vi "test_read-nmea-data2.vi"() -> ()   [LabVIEW 2019] (continued)
32,154,14,19,51,157,,6*69\n\t\n15:14:47.48\tF9P\t$GPGSV,3,3,09,25,12,306,,6*5B\n\t\n15:14:47.50\tF9P\t$GLGSV,2,1,08,69,10,031,33,70,70,037,27,71,54,207,28,72,05,210,,1*75\n\t\n15:14:47.52\tF9P\t$GLGSV,2,2,08,77,01,324,,84,19,123,21,85,69,072,36,86,38,331,,1*75\n\t\n15:14:47.54\tF9P\t$GLGSV,2,1,08,69,10,031,20,70,70,037,,71,54,207,24,72,05,210,,3*7C\n\t\n15:14:47.56\tF9P\t$GLGSV,2,2,08,77,01,324,,84,19,123,27,85,69,072,25,86,38,331,,3*73\n\t\n15:14:47.58\tF9P\t$GAGSV,2,1,08,02,08,296,09,04,67,115,26,09,33,193,34,11,72,001,24,7*75\n\t\n15:14:47.60\tF9P\t$GAGSV,2,2,08,12,39,103,28,19,25,045,35,25,08,248,21,36,27,309,18,7*73\n\t\n15:14:47.62\tF9P\t$GAGSV,2,1,08,02,08,296,,04,67,115,24,09,33,193,,11,72,001,,2*7A\n\t\n15:14:47.64\tF9P\t$GAGSV,2,2,08,12,39,103,,19,25,045,,25,08,248,,36,27,309,,2*70\n\t\n15:14:47.66\tF9P\t$GBGSV,2,1,06,07,,,24,11,48,133,32,14,87,101,26,28,,,26,1*7E\n\t\n15:14:47.68\tF9P\t$GBGSV,2,2,06,33,62,220,30,34,,,40,1*44\n\t\n15:14:47.70\tF9P\t$GBGSV,1,1,03,11,48,133,25,14,87,101,,33,62,220,,3*43\n\t\n15:14:47.72\tF9P\t$GNGLL,3723.60420,N,12656.96638,E,061449.00,A,A*78\n\t\n15:14:47.74\tF9P\t\t\n15:14:47.76\tF9P\t\t\n15:14:47.78\tF9P\t\t\n15:14:47.80\tF9P\t\t\n15:14:47.82\tF9P\t\t\n15:14:47.84\tF9P\t\t\n15:14:47.86\tF9P\t\t\n15:14:47.88\tF9P\t\t\n15:14:47.90\tF9P\t\t\n15:14:47.92\tF9P\t\t\n15:14:47.94\tF9P\t\t\n15:14:47.96\tF9P\t\t\n15:14:47.98\tF9P\t\t\n15:14:48.00\tF9P\t\t\n15:14:48.02\tF9P\t\t\n15:14:48.04\tF9P\t\t\n15:14:48.06\tF9P\t\t\n15:14:48.08\tF9P\t\t\n15:14:48.10\tF9P\t\t\n15:14:48.12\tF9P\t\t\n15:14:48.14\tF9P\t\t\n15:14:48.16\tF9P\t\t\n15:14:48.18\tF9P\t\t\n15:14:48.20\tF9P\t\t\n15:14:48.22\tF9P\t\t\n15:14:48.24\tF9P\t$GNRMC,061450.00,A,3723.60390,N,12656.96564,E,2.579,234.40,250720,,,A,V*01\n\t\n15:14:48.26\tF9P\t$GNVTG,234.40,T,,M,2.579,N,4.776,K,A*29\n\t\n15:14:48.28\tF9P\t$GNGGA,061450.00,3723.60390,N,12656.96564,E,1,12,0.64,46.4,M,18.5,M,,*78\n\t\n15:14:48.30\tF9P\t$GNGSA,A,3,12,06,19,05,17,09,04,02,,,,,1.14,0.64,0.95,1*0A\n\t\n15:14:48.32\tF9P\t$GNGSA,A,3,85,70,71,84,,,,,,,,,1.14,0.64,0.95,2*08\n\t\n15:14:48.34\tF9P\t$GNGSA,A,3,36,19,11,04,09,12,,,,,,,1.14,0.64,0.95,3*0A\n\t\n15:14:48.36\tF9P\t$GNGSA,A,3,14,11,33,,,,,,,,,,1.14,0.64,0.95,4*0B\n\t\n15:14:48.38\tF9P\t$GPGSV,3,1,09,02,56,320,22,04,17,043,37,05,38,248,32,06,64,051,35,1*69\n\t\n15:14:48.40\tF9P\t$GPGSV,3,2,09,09,44,073,41,12,23,276,25,17,32,154,28,19,51,157,32,1*61\n\t\n15:14:48.42\tF9P\t$GPGSV,3,3,09,25,12,306,15,1*58\n\t\n15:14:48.44\tF9P\t$GPGSV,3,1,09,02,56,320,,04,17,043,23,05,38,248,17,06,64,051,27,6*6F\n\t\n15:14:48.46\tF9P\t$GPGSV,3,2,09,09,44,073,27,12,23,276,16,17,32,154,14,19,51,157,,6*68\n\t\n15:14:48.48\tF9P\t$GPGSV,3,3,09,25,12,306,,6*5B\n\t\n15:14:48.50\tF9P\t$GLGSV,2,1,08,69,10,031,28,70,70,037,27,71,54,207,32,72,05,210,,1*74\n\t\n15:14:48.52\tF9P\t$GLGSV,2,2,08,77,01,324,,84,19,123,21,85,69,072,35,86,38,331,,1*76\n\t\n15:14:48.54\tF9P\t$GLGSV,2,1,08,69,10,031,20,70,70,037,,71,54,207,23,72,05,210,,3*7B\n\t\n15:14:48.56\tF9P\t$GLGSV,2,2,08,77,01,324,,84,19,123,27,85,69,072,23,86,38,331,,3*75\n\t\n15:14:48.58\tF9P\t$GAGSV,2,1,08,02,08,296,12,04,67,115,32,09,33,193,30,11,72,001,25,7*7F\n\t\n15:14:48.60\tF9P\t$GAGSV,2,2,08,12,39,103,28,19,25,045,34,25,08,248,21,36,27,309,18,7*72\n\t\n15:14:48.62\tF9P\t$GAGSV,2,1,08,02,08,296,,04,67,115,,09,33,193,,11,72,001,,2*7C\n\t\n15:14:48.64\tF9P\t$GAGSV,2,2,08,12,39,103,,19,25,045,,25,08,248,,36,27,309,,2*70\n\t\n15:14:48.66\tF9P\t$GBGSV,2,1,06,07,,,26,11,48,133,40,14,87,101,27,28,,,25,1*7B\n\t\n15:14:48.68\tF9P\t$GBGSV,2,2,06,33,62,220,33,34,,,25,1*44\n\t\n15:14:48.70\tF9P\t$GBGSV,1,1,03,11,48,133,24,14,87,101,27,33,62,220,,3*47\n\t\n15:14:48.72\tF9P\t$GNGLL,3723.60390,N,12656.96564,E,061450.00,A,A*76\n\t\n15:14:48.74\tF9P\t\t\n15:14:48.76\tF9P\t\t\n15:14:48.78\tF9P\t\t\n15:14:48.80\tF9P\t\t\n15:14:48.82\tF9P\t\t\n15:14:48.84\tF9P\t\t\n15:14:48.86\tF9P\t\t\n15:14:48.88\tF9P\t\t\n15:14:48.90\tF9P\t\t\n15:14:48.92\tF9P\t\t\n15:14:48.94\tF9P\t\t\n15:14:48.96\tF9P\t\t\n15:14:48.98\tF9P\t\t\n15:14:49.00\tF9P\t\t\n15:14:49.02\tF9P\t\t\n15:14:49.04\tF9P\t\t\n15:14:49.06\tF9P\t\t\n15:14:49.08\tF9P\t\t\n15:14:49.10\tF9P\t\t\n15:14:49.12\tF9P\t\t\n15:14:49.14\tF9P\t\t\n15:14:49.16\tF9P\t\t\n15:14:49.18\tF9P\t\t\n15:14:49.20\tF9P\t\t\n15:14:49.22\tF9P\t\t\n15:14:49.24\tF9P\t$GNRMC,061451.00,A,3723.60369,N,12656.96492,E,2.264,236.00,250720,,,A,V*03\n\t\n15:14:49.26\tF9P\t$GNVTG,236.00,T,,M,2.264,N,4.193,K,A*29\n\t\n15:14:49.28\tF9P\t$GNGGA,061451.00,3723.60369,N,12656.96492,E,1,12,0.70,46.7,M,18.5,M,,*71\n\t\n15:14:49.30\tF9P\t$GNGSA,A,3,12,06,19,05,17,09,04,02,,,,,1.23,0.70,1.01,1*07\n\t\n15:14:49.32\tF9P\t$GNGSA,A,3,85,70,71,84,,,,,,,,,1.23,0.70,1.01,2*05\n\t\n15:14:49.34\tF9P\t$GNGSA,A,3,36,19,11,04,09,12,,,,,,,1.23,0.70,1.01,3*07\n\t\n15:14:49.36\tF9P\t$GNGSA,A,3,14,11,33,,,,,,,,,,1.23,0.70,1.01,4*06\n\t\n15:14:49.38\tF9P\t$GPGSV,3,1,09,02,56,320,22,04,17,043,30,05,38,248,35,06,64,051,30,1*6C\n\t\n15:14:49.40\tF9P\t$GPGSV,3,2,09,09,44,073,35,12,23,276,25,17,32,154,27,19,51,157,27,1*69\n\t\n15:14:49.42\tF9P\t$GPGSV,3,3,09,25,12,306,13,1*5E\n\t\n15:14:49.44\tF9P\t$GPGSV,3,1,09,02,56,320,,04,17,043,24,05,38,248,28,06,64,051,27,6*64\n\t\n15:14:49.46\tF9P\t$GPGSV,3,2,09,09,44,073,27,12,23,276,16,17,32,154,13,19,51,157,,6*6F\n\t\n15:14:49.48\tF9P\t$GPGSV,3,3,09,25,12,306,,6*5B\n\t\n15:14:49.50\tF9P\t$GLGSV,2,1,08,69,10,031,27,70,70,037,35,71,54,207,29,72,05,210,,1*72\n\t\n15:14:49.52\tF9P\t$GLGSV,2,2,08,77,01,324,,84,19,123,22,85,69,072,37,86,38,331,,1*77\n\t\n15:14:49.54\tF9P\t$GLGSV,2,1,08,69,10,031,19,70,70,037,,71,54,207,23,72,05,210,,3*71\n\t\n15:14:49.56\tF9P\t$GLGSV,2,2,08,77,01,324,,84,19,123,32,85,69,072,23,86,38,331,,3*71\n\t\n15:14:49.58\tF9P\t$GAGSV,2,1,08,02,08,296,10,04,67,115,27,09,33,193,24,11,72,001,25,7*7C\n\t\n15:14:49.60\tF9P\t$GAGSV,2,2,08,12,39,103,27,19,25,045,33,25,08,248,20,36,27,309,19,7*7A\n\t\n15:14:49.62\tF9P\t$GAGSV,2,1,08,02,08,296,,04,67,115,,09,33,193,,11,72,001,,2*7C\n\t\n15:14:49.64\tF9P\t$GAGSV,2,2,08,12,39,103,,19,25,045,,25,08,248,,36,27,309,,2*70\n\t\n15:14:49.66\tF9P\t$GBGSV,2,1,06,07,,,28,11,48,133,27,14,87,101,31,28,,,24,1*72\n\t\n15:14:49.68\tF9P\t$GBGSV,2,2,06,33,62,220,36,34,,,27,1*43\n\t\n15:14:49.70\tF9P\t$GBGSV,1,1,03,11,48,133,23,14,87,101,30,33,62,220,,3*46\n\t\n15:14:49.72\tF9P\t$GNGLL,3723.60369,N,12656.96492,E,061451.00,A,A*79\n\t\n15:14:49.74\tF9P\t\t\n15:14:49.76\tF9P\t\t\n15:14:49.78\tF9P\t\t\n15:14:49.80\tF9P\t\t\n15:14:49.82\tF9P\t\t\n15:14:49.84\tF9P\t\t\n15:14:49.86\tF9P\t\t\n15:14:49.88\tF9P\t\t\n15:14:49.90\tF9P\t\t\n15:14:49.92\tF9P\t\t\n15:14:49.94\tF9P\t\t\n15:14:49.96\tF9P\t\t\n15:14:49.98\tF9P\t\t\n15:14:50.00\tF9P\t\t\n15:14:50.02\tF9P\t\t\n15:14:50.04\tF9P\t\t\n15:14:50.06\tF9P\t\t\n15:14:50.08\tF9P\t\t\n15:14:50.10\tF9P\t\t\n15:14:50.12\tF9P\t\t\n15:14:50.14\tF9P\t\t\n15:14:50.16\tF9P\t\t\n15:14:50.18\tF9P\t\t\n15:14:50.20\tF9P\t\t\n15:14:50.22\tF9P\t\t\n15:14:50.24\tF9P\t$GNRMC,061452.00,A,3723.60353,N,12656.96391,E,2.556,238.12,250720,,,A,V*06\n\t\n15:14:50.26\tF9P\t$GNVTG,238.12,T,,M,2.556,N,4.734,K,A*29\n\t\n15:14:50.28\tF9P\t$GNGGA,061452.00,3723.60353,N,12656.96391,E,1,12,0.69,46.6,M,18.5,M,,*76\n\t\n15:14:50.30\tF9P\t$GNGSA,A,3,12,06,19,05,17,09,04,02,,,,,1.20,0.69,0.98,1*0D\n\t\n15:14:50.32\tF9P\t$GNGSA,A,3,85,70,71,84,,,,,,,,,1.20,0.69,0.98,2*0F\n\t\n15:14:50.34\tF9P\t$GNGSA,A,3,36,19,11,04,09,12,,,,,,,1.20,0.69,0.98,3*0D\n\t\n15:14:50.36\tF9P\t$GNGSA,A,3,14,11,33,,,,,,,,,,1.20,0.69,0.98,4*0C\n\t\n15:14:50.38\tF9P\t$GPGSV,3,1,09,02,56,320,22,04,17,043,36,05,38,248,36,06,64,051,31,1*68\n\t\n15:14:50.40\tF9P\t$GPGSV,3,2,09,09,44,073,35,12,23,276,24,17,32,154,32,19,51,157,31,1*6B\n\t\n15:14:50.42\tF9P\t$GPGSV,3,3,09,25,12,306,12,1*5F\n\t\n15:14:50.44\tF9P\t$GPGSV,3,1,09,02,56,320,,04,17,043,24,05,38,248,27,06,64,051,32,6*6F\n\t\n15:14:50.46\tF9P\t$GPGSV,3,2,09,09,44,073,27,12,23,276,14,17,32,154,14,19,51,157,,6*6A\n\t\n15:14:50.48\tF9P\t$GPGSV,3,3,09,25,12,306,,6*5B\n\t\n15:14:50.50\tF9P\t$GLGSV,2,1,08,69,10,031,31,70,70,037,32,71,54,207,30,72,05,210,,1*7A\n\t\n15:14:50.52\tF9P\t$GLGSV,2,2,08,77,01,324,,84,19,123,23,85,69,072,41,86,38,331,,1*77\n\t\n15:14:50.54\tF9P\t$GLGSV,2,1,08,69,10,031,19,70,70,037,,71,54,207,24,72,05,210,,3*76\n\t\n15:14:50.56\tF9P\t$GLGSV,2,2,08,77,01,324,,84,19,123,37,85,69,072,23,86,38,331,,3*74\n\t\n15:14:50.58\tF9P\t$GAGSV,2,1,08,02,08,296,11,04,67,115,30,09,33,193,30,11,72,001,24,7*7F\n\t\n15:14:50.60\tF9P\t$GAGSV,2,2,08,12,39,103,31,19,25,045,29,25,08,248,19,36,27,309,19,7*7C\n\t\n15:14:50.62\tF9P\t$GAGSV,2,1,08,02,08,296,,04,67,115,,09,33,193,,11,72,001,,2*7C\n\t\n15:14:50.64\tF9P\t$GAGSV,2,2,08,12,39,103,,19,25,045,,25,08,248,,36,27,309,,2*70\n\t\n15:14:50.66\tF9P\t$GBGSV,2,1,06,07,,,30,11,48,133,26,14,87,101,34,28,,,23,1*78\n\t\n15:14:50.68\tF9P\t$GBGSV,2,2,06,33,62,220,35,34,,,25,1*42\n\t\n15:14:50.70\tF9P\t$GBGSV,1,1,03,11,48,133,28,14,87,101,33,33,62,220,,3*4E\n\t\n15:14:50.72\tF9P\t$GNGLL,3723.60353,N,12656.96391,E,061452.00,A,A*77\n\t\n15:14:50.74\tF9P\t\t\n15:14:50.76\tF9P\t\t\n15:14:50.78\tF9P\t\t\n15:14:50.80\tF9P\t\t\n15:14:50.82\tF9P\t\t\n15:14:50.84\tF9P\t\t\n15:14:50.86\tF9P\t\t\n15:14:50.88\tF9P\t\t\n15:14:50.90\tF9P\t\t\n15:14:50.92\tF9P\t\t\n15:14:50.94\tF9P\t\t\n15:14:50.96\tF9P\t\t\n15:14:50.98\tF9P\t\t\n15:14:51.00\tF9P\t\t\n15:14:51.02\tF9P\t\t\n15:14:51.04\tF9P\t\t\n15:14:51.06\tF9P\t\t\n15:14:51.08\tF9P\t\t\n15:14:51.10\tF9P\t\t\n15:14:51.12\tF9P\t\t\n15:14:51.14\tF9P\t\t\n15:14:51.16\tF9P\t\t\n15:14:51.18\tF9P\t\t\n15:14:51.20\tF9P\t\t\n15:14:51.22\tF9P\t\t\n15:14:51.24\tF9P\t$GNRMC,061453.00,A,3723.60346,N,12656.96277,E,2.685,246.04,250720,,,A,V*09\n\t\n15:14:51.26\tF9P\t$GNVTG,246.04,T,,M,2.685,N,4.973,K,A*27\n\t\n15:14:51.28\tF9P\t$GNGGA,061453.00,3723.60346,N,12656.96277,E,1,12,0.72,46.9,M,18.5,M,,*7F\n\t\n15:14:51.30\tF9P\t$GNGSA,A,3,12,06,19,05,17,09,04,02,,,,,1.24,0.72,1.01,1*02\n\t\n15:14:51.32\tF9P\t$GNGSA,A,3,85,70,71,84,,,,,,,,,1.24,0.72,1.01,2*00\n\t\n15:14:51.34\tF9P\t$GNGSA,A,3,36,19,11,04,09,12,,,,,,,1.24,0.72,1.01,3*02\n\t\n15:14:51.36\tF9P\t$GNGSA,A,3,14,11,33,,,,,,,,,,1.24,0.72,1.01,4*03\n\t\n15:14:51.38\tF9P\t$GPGSV,3,1,09,02,56,320,23,04,17,043,33,05,38,248,36,06,64,051,32,1*6F\n\t\n15:14:51.40\tF9P\t$GPGSV,3,2,09,09,44,072,38,12,23,276,24,17,32,154,27,19,51,157,25,1*66\n\t\n15:14:51.42\tF9P\t$GPGSV,3,3,09,25,12,306,11,1*5C\n\t\n15:14:51.44\tF9P\t$GPGSV,3,1,09,02,56,320,,04,17,043,23,05,38,248,33,06,64,051,32,6*6D\n\t\n15:14:51.46\tF9P\t$GPGSV,3,2,09,09,44,072,32,12,23,276,12,17,32,154,15,19,51,157,,6*68\n\t\n15:14:51.48\tF9P\t$GPGSV,3,3,09,25,12,306,,6*5B\n\t\n15:14:51.50\tF9P\t$GLGSV,2,1,08,69,10,031,27,70,70,037,27,71,54,207,30,72,05,210,,1*79\n\t\n15:14:51.52\tF9P\t$GLGSV,2,2,08,77,01,324,,84,19,123,23,85,69,072,39,86,38,331,,1*78\n\t\n15:14:51.54\tF9P\t$GLGSV,2,1,08,69,10,031,19,70,70,037,,71,54,207,24,72,05,210,,3*76\n\t\n15:14:51.56\tF9P\t$GLGSV,2,2,08,77,01,324,,84,19,123,31,85,69,072,23,86,38,331,,3*72\n\t\n15:14:51.58\tF9P\t$GAGSV,2,1,08,02,08,296,07,04,67,115,31,09,33,193,28,11,72,001,24,7*70\n\t\n15:14:51.60\tF9P\t$GAGSV,2,2,08,12,39,103,22,19,25,045,30,25,08,248,15,36,27,309,18,7*7B\n\t\n15:14:51.62\tF9P\t$GAGSV,2,1,08,02,08,296,,04,67,115,,09,33,193,,11,72,001,,2*7C\n\t\n15:14:51.64\tF9P\t$GAGSV,2,2,08,12,39,103,,19,25,045,,25,08,248,,36,27,309,,2*70\n\t\n15:14:51.66\tF9P\t$GBGSV,2,1,06,07,,,33,11,48,133,27,14,87,101,34,28,,,22,1*7B\n\t\n15:14:51.68\tF9P\t$GBGSV,2,2,06,33,62,220,32,34,,,25,1*45\n\t\n15:14:51.70\tF9P\t$GBGSV,1,1,03,11,48,133,25,14,87,101,32,33,62,220,,3*42\n\t\n15:14:51.72\tF9P\t$GNGLL,3723.60346,N,12656.96277,E,061453.00,A,A*7B\n\t\n15:14:51.74\tF9P\t\t\n15:14:51.76\tF9P\t\t\n15:14:51.78\tF9P\t\t\n15:14:51.80\tF9P\t\t\n15:14:51.82\tF9P\t\t\n15:14:51.84\tF9P\t\t\n15:14:51.86\tF9P\t\t\n15:14:51.88\tF9P\t\t\n15:14:51.90\tF9P\t\t\n15:14:51.92\tF9P\t\t\n15:14:51.94\tF9P\t\t\n15:14:51.96\tF9P\t\t\n15:14:51.98\tF9P\t\t\n15:14:52.00\tF9P\t\t\n15:14:52.02\tF9P\t\t\n15:14:52.04\tF9P\t\t\n15:14:52.06\tF9P\t\t\n15:14:52.08\tF9P\t\t\n15:14:52.10\tF9P\t\t\n15:14:52.12\tF9P\t\t\n15:14:52.14\tF9P\t\t\n15:14:52.16\tF9P\t\t\n15:14:52.18\tF9P\t\t\n15:14:52.20\tF9P\t\t\n15:14:52.22\tF9P\t\t\n15:14:52.24\tF9P\t$GNRMC,061454.00,A,3723.60329,N,12656.96190,E,2.545,245.64,250720,,,A,V*07\n\t\n15:14:52.26\tF9P\t$GNVTG,245.64,T,,M,2.545,N,4.712,K,A*24\n\t\n15:14:52.28\tF9P\t$GNGGA,061454.00,3723.60329,N,12656.96190,E,1,12,0.69,46.9,M,18.5,M,,*71\n\t\n15:14:52.30\tF9P\t$GNGSA,A,3,12,06,19,05,17,09,04,02,,,,,1.20,0.69,0.98,1*0D\n\t\n15:14:52.32\tF9P\t$GNGSA,A,3,85,70,71,84,,,,,,,,,1.20,0.69,0.98,2*0F\n\t\n15:14:52.34\tF9P\t$GNGSA,A,3,36,19,11,04,09,12,,,,,,,1.20,0.69,0.98,3*0D\n\t\n15:14:52.36\tF9P\t$GNGSA,A,3,14,11,33,,,,,,,,,,1.20,0.69,0.98,4*0C\n\t\n15:14:52.38\tF9P\t$GPGSV,3,1,09,02,56,320,25,04,17,043,28,05,38,248,36,06,64,051,28,1*68\n\t\n15:14:52.40\tF9P\t$GPGSV,3,2,09,09,44,072,31,12,23,276,23,17,32,154,27,19,51,157,25,1*68\n\t\n15:14:52.42\tF9P\t$GPGSV,3,3,09,25,12,306,12,1*5F\n\t\n15:14:52.44\tF9P\t$GPGSV,3,1,09,02,56,320,,04,17,043,21,05,38,248,35,06,64,051,32,6*69\n\t\n15:14:52.46\tF9P\t$GPGSV,3,2,09,09,44,072,28,12,23,276,17,17,32,154,16,19,51,157,,6*65\n\t\n15:14:52.48\tF9P\t$GPGSV,3,3,09,25,12,306,,6*5B\n\t\n15:14:52.50\tF9P\t$GLGSV,2,1,08,69,10,031,26,70,70,037,28,71,54,207,31,72,05,210,,1*76\n\t\n15:14:52.52\tF9P\t$GLGSV,2,2,08,77,01,324,,84,19,123,23,85,69,072,41,86,38,331,,1*77\n\t\n15:14:52.54\tF9P\t$GLGSV,2,1,08,69,10,031,19,70,70,037,,71,54,207,26,72,05,210,,3*74\n\t\n15:14:52.56\tF9P\t$GLGSV,2,2,08,77,01,324,,84,19,123,30,85,69,072,25,86,38,331,,3*75\n\t\n15:14:52.58\tF9P\t$GAGSV,2,1,08,02,08,296,12,04,67,115,28,09,33,193,32,11,72,001,24,7*77\n\t\n15:14:52.60\tF9P\t$GAGSV,2,2,08,12,39,103,23,19,25,045,34,25,08,248,14,36,27,309,18,7*7F\n\t\n15:14:52.62\tF9P\t$GAGSV,2,1,08,02,08,296,,04,67,115,,09,33,193,,11,72,001,,2*7C\n\t\n15:14:52.64\tF9P\t$GAGSV,2,2,08,12,39,103,,19,25,045,,25,08,248,,36,27,309,,2*70\n\t\n15:14:52.66\tF9P\t$GBGSV,2,1,06,07,,,33,11,48,133,26,14,87,101,31,28,,,23,1*7E\n\t\n15:14:52.68\tF9P\t$GBGSV,2,2,06,33,62,220,32,34,,,25,1*45\n\t\n15:14:52.70\tF9P\t$GBGSV,1,1,03,11,48,133,24,14,87,101,29,33,62,220,,3*49\n\t\n15:14:52.72\tF9P\t$GNGLL,3723.60329,N,12656.96190,E,061454.00,A,A*7F\n\t\n15:14:52.74\tF9P\t\t\n15:14:52.76\tF9P\t\t\n15:14:52.78\tF9P\t\t\n15:14:52.80\tF9P\t\t\n15:14:52.82\tF9P\t\t\n15:14:52.84\tF9P\t\t\n15:14:52.86\tF9P\t\t\n15:14:52.88\tF9P\t\t\n15:14:52.90\tF9P\t\t\n15:14:52.92\tF9P\t\t\n15:14:52.94\tF9P\t\t\n15:14:52.96\tF9P\t\t\n15:14:52.98\tF9P\t\t\n15:14:53.00\tF9P\t\t\n15:14:53.02\tF9P\t\t\n15:14:53.04\tF9P\t\t\n15:14:53.06\tF9P\t\t\n15:14:53.08\tF9P\t\t\n15:14:53.10\tF9P\t\t\n15:14:53.12\tF9P\t\t\n15:14:53.14\tF9P\t\t\n15:14:53.16\tF9P\t\t\n15:14:53.18\tF9P\t\t\n15:14:53.20\tF9P\t\t\n15:14:53.22\tF9P\t\t\n15:14:53.24\tF9P\t$GNRMC,061455.00,A,3723.60312,N,12656.96092,E,2.849,246.15,250720,,,A,V*09\n\t\n15:14:53.26\tF9P\t$GNVTG,246.15,T,,M,2.849,N,5.277,K,A*27\n\t\n15:14:53.28\tF9P\t$GNGGA,061455.00,3723.60312,N,12656.96092,E,1,12,0.72,46.5,M,18.5,M,,*7D\n\t\n15:14:53.30\tF9P\t$GNGSA,A,3,12,06,19,05,17,09,04,02,,,,,1.24,0.72,1.01,1*02\n\t\n15:14:53.32\tF9P\t$GNGSA,A,3,85,70,71,84,,,,,,,,,1.24,0.72,1.01,2*00\n\t\n15:14:53.34\tF9P\t$GNGSA,A,3,36,19,11,04,09,12,,,,,,,1.24,0.72,1.01,3*02\n\t\n15:14:53.36\tF9P\t$GNGSA,A,3,14,11,33,,,,,,,,,,1.24,0.72,1.01,4*03\n\t\n15:14:53.38\tF9P\t$GPGSV,3,1,09,02,56,320,30,04,17,043,33,05,38,248,34,06,64,051,38,1*65\n\t\n15:14:53.40\tF9P\t$GPGSV,3,2,09,09,44,072,38,12,23,276,23,17,32,154,27,19,51,157,25,1*61\n\t\n15:14:53.42\tF9P\t$GPGSV,3,3,09,25,12,306,14,1*59\n\t\n15:14:53.44\tF9P\t$GPGSV,3,1,09,02,56,320,,04,17,043,22,05,38,248,27,06,64,051,31,6*6A\n\t\n15:14:53.46\tF9P\t$GPGSV,3,2,09,09,44,072,27,12,23,276,19,17,32,154,17,19,51,157,,6*65\n\t\n15:14:53.48\tF9P\t$GPGSV,3,3,09,25,12,306,,6*5B\n\t\n15:14:53.50\tF9P\t$GLGSV,2,1,08,69,10,031,26,70,70,037,34,71,54,207,36,72,05,210,,1*7C\n\t\n15:14:53.52\tF9P\t$GLGSV,2,2,08,77,01,324,,84,19,123,21,85,69,072,42,86,38,331,,1*76\n\t\n15:14:53.54\tF9P\t$GLGSV,2,1,08,69,10,031,19,70,70,037,,71,54,207,24,72,05,210,,3*76\n\t\n15:14:53.56\tF9P\t$GLGSV,2,2,08,77,01,324,,84,19,123,23,85,69,072,26,86,38,331,,3*74\n\t\n15:14:53.58\tF9P\t$GAGSV,2,1,08,02,08,296,11,04,67,115,33,09,33,193,27,11,72,001,22,7*7C\n\t\n15:14:53.60\tF9P\t$GAGSV,2,2,08,12,39,103,27,19,25,045,33,25,08,248,12,36,27,309,18,7*7A\n\t\n15:14:53.62\tF9P\t$GAGSV,2,1,08,02,08,296,,04,67,115,,09,33,193,,11,72,001,,2*7C\n\t\n15:14:53.64\tF9P\t$GAGSV,2,2,08,12,39,103,,19,25,045,,25,08,248,,36,27,309,,2*70\n\t\n15:14:53.66\tF9P\t$GBGSV,2,1,06,07,,,28,11,48,133,26,14,87,101,34,28,,,23,1*71\n\t\n15:14:53.68\tF9P\t$GBGSV,2,2,06,33,62,220,28,34,,,25,1*4E\n\t\n15:14:53.70\tF9P\t$GBGSV,1,1,03,11,48,133,,14,87,101,28,33,62,220,,3*4E\n\t\n15:14:53.72\tF9P\t$GNGLL,3723.60312,N,12656.96092,E,061455.00,A,A*75\n\t\n15:14:53.74\tF9P\t\t\n15:14:53.76\tF9P\t\t\n15:14:53.78\tF9P\t\t\n15:14:53.80\tF9P\t\t\n15:14:53.82\tF9P\t\t\n15:14:53.84\tF9P\t\t\n15:14:53.86\tF9P\t\t\n15:14:53.88\tF9P\t\t\n15:14:53.90\tF9P\t\t\n15:14:53.92\tF9P\t\t\n15:14:53.94\tF9P\t\t\n15:14:53.97\tF9P\t\t\n15:14:53.99\tF9P\t\t\n15:14:54.01\tF9P\t\t\n15:14:54.03\tF9P\t\t\n15:14:54.05\tF9P\t\t\n15:14:54.07\tF9P\t\t\n15:14:54.09\tF9P\t\t\n15:14:54.11\tF9P\t\t\n15:14:54.13\tF9P\t\t\n15:14:54.15\tF9P\t\t\n15:14:54.17\tF9P\t\t\n15:14:54.19\tF9P\t\t\n15:14:54.21\tF9P\t\t\n15:14:54.23\tF9P\t$GNRMC,061456.00,A,3723.60295,N,12656.96011,E,2.274,243.02,25072\t\n15:14:54.25\tF9P\t0,,,A,V*08\n\t\n15:14:54.27\tF9P\t$GNVTG,243.02,T,,M,2.274,N,4.211,K,A*21\n\t\n15:14:54.29\tF9P\t$GNGGA,061456.00,3723.60295,N,12656.96011,E,1,12,0.70,45.8,M,18.5,M,,*77\n\t\n15:14:54.31\tF9P\t$GNGSA,A,3,12,06,19,05,17,09,04,02,,,,,1.23,0.70,1.01,1*07\n\t\n15:14:54.33\tF9P\t$GNGSA,A,3,85,70,71,84,,,,,,,,,1.23,0.70,1.01,2*05\n\t\n15:14:54.35\tF9P\t$GNGSA,A,3,36,19,11,04,09,12,,,,,,,1.23,0.70,1.01,3*07\n\t\n15:14:54.37\tF9P\t$GNGSA,A,3,14,11,33,,,,,,,,,,1.23,0.70,1.01,4*06\n\t\n15:14:54.39\tF9P\t$GPGSV,3,1,09,02,56,320,28,04,17,043,33,05,38,248,34,06,64,051,30,1*64\n\t\n15:14:54.41\tF9P\t$GPGSV,3,2,09,09,44,072,38,12,23,275,24,17,32,154,27,19,51,157,31,1*60\n\t\n15:14:54.43\tF9P\t$GPGSV,3,3,09,25,12,306,15,1*58\n\t\n15:14:54.45\tF9P\t$GPGSV,3,1,09,02,56,320,,04,17,043,20,05,38,248,27,06,64,051,26,6*6E\n\t\n15:14:54.47\tF9P\t$GPGSV,3,2,09,09,44,072,28,12,23,275,17,17,32,154,15,19,51,157,,6*65\n\t\n15:14:54.49\tF9P\t$GPGSV,3,3,09,25,12,306,,6*5B\n\t\n15:14:54.51\tF9P\t$GLGSV,2,1,08,69,10,031,25,70,70,037,29,71,54,207,36,72,05,210,,1*73\n\t\n15:14:54.53\tF9P\t$GLGSV,2,2,08,77,01,324,,84,19,123,20,85,69,072,41,86,38,331,,1*74\n\t\n15:14:54.55\tF9P\t$GLGSV,2,1,08,69,10,031,19,70,70,037,,71,54,207,24,72,05,210,,3*76\n\t\n15:14:54.57\tF9P\t$GLGSV,2,2,08,77,01,324,,84,19,123,22,85,69,072,26,86,38,331,,3*75\n\t\n15:14:54.59\tF9P\t$GAGSV,2,1,08,02,08,296,09,04,67,115,35,09,33,193,32,11,72,001,23,7*76\n\t\n15:14:54.61\tF9P\t$GAGSV,2,2,08,12,39,103,32,19,25,045,37,25,08,248,12,36,27,309,20,7*71\n\t\n15:14:54.63\tF9P\t$GAGSV,2,1,08,02,08,296,,04,67,115,28,09,33,193,,11,72,001,,2*76\n\t\n15:14:54.65\tF9P\t$GAGSV,2,2,08,12,39,103,,19,25,045,,25,08,248,,36,27,309,,2*70\n\t\n15:14:54.67\tF9P\t$GBGSV,2,1,06,07,,,28,11,48,133,26,14,87,101,34,28,,,23,1*71\n\t\n15:14:54.69\tF9P\t$GBGSV,2,2,06,33,62,220,29,34,,,25,1*4F\n\t\n15:14:54.71\tF9P\t$GBGSV,1,1,03,11,48,133,,14,87,101,32,33,62,220,,3*45\n\t\n15:14:54.73\tF9P\t$GNGLL,3723.60295,N,12656.96011,E,061456.00,A,A*73\n\t\n15:14:54.75\tF9P\t\t\n15:14:54.77\tF9P\t\t\n15:14:54.79\tF9P\t\t\n15:14:54.81\tF9P\t\t\n15:14:54.83\tF9P\t\t\n15:14:54.85\tF9P\t\t\n15:14:54.87\tF9P\t\t\n15:14:54.89\tF9P\t\t\n15:14:54.91\tF9P\t\t\n15:14:54.93\tF9P\t\t\n15:14:54.95\tF9P\t\t\n15:14:54.97\tF9P\t\t\n15:14:54.99\tF9P\t\t\n15:14:55.01\tF9P\t\t\n15:14:55.03\tF9P\t\t\n15:14:55.05\tF9P\t\t\n15:14:55.07\tF9P\t\t\n15:14:55.09\tF9P\t\t\n15:14:55.11\tF9P\t\t\n15:14:55.13\tF9P\t\t\n15:14:55.15\tF9P\t\t\n15:14:55.17\tF9P\t\t\n15:14:55.19\tF9P\t\t\n15:14:55.21\tF9P\t\t\n15:14:55.23\tF9P\t$GNRMC,061457.00,A,3723.60262,N,12656.95923
